vi "Excel Inert Image.vi"(4 "Cell/表格位置2":string, 6 "Cell/表格位置1":string, 8 "错误输入":errorcluster, 9 "图片路径":path, 11 "Excel._Worksheet in":refnum<k7>) -> (0 "错误输出":errorcluster, 2 "AddPicture":refnum<k7>, 3 "Excel._Worksheet out":refnum<k7>)   [LabVIEW 2011]
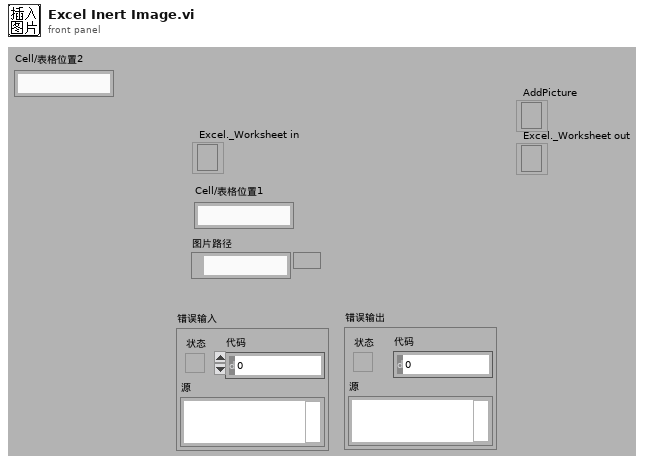
[diagram p1: front panel]
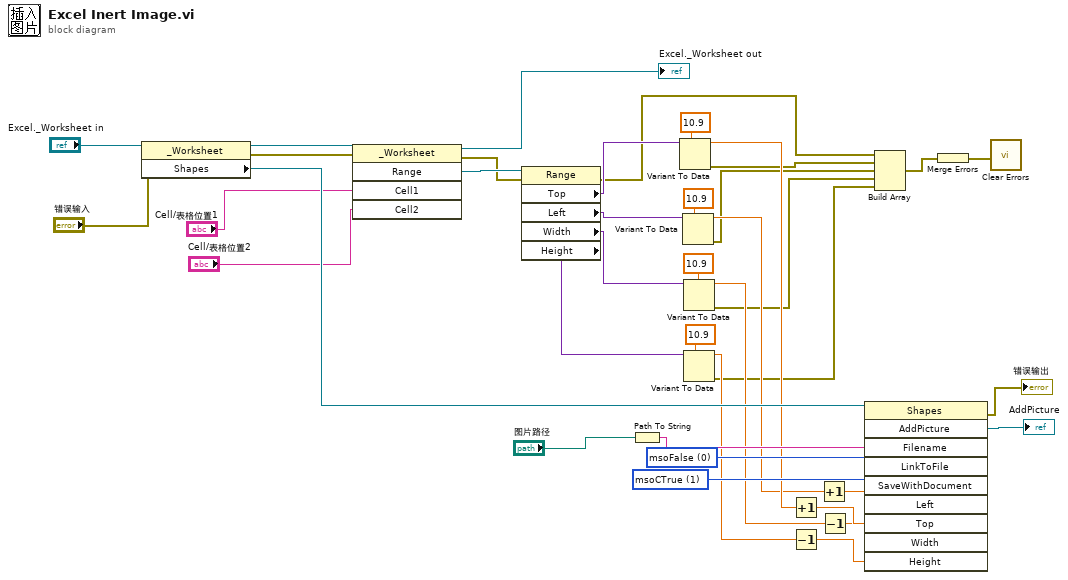
[diagram p0: block diagram]
diagram:
  w33 = 1 items=["msoTrue"=-1, "msoFalse"=0, "msoCTrue"=1, "msoTriStateToggle"=-3, "msoTriStateMixed"=-2] ("SaveWithDocument")
  w34 = 0 items=["msoTrue"=-1, "msoFalse"=0, "msoCTrue"=1, "msoTriStateToggle"=-3, "msoTriStateMixed"=-2] ("LinkToFile")
  n1 = property class="_Worksheet"(reference="Excel._Worksheet in", error in="错误输入") -> (reference out=w39:refnum<k7>, error out=w37:errorcluster, "Shapes"=w38:refnum<k7>)
  n2 = invoke class="_Worksheet" method="Range"(reference=w39, error in=w37, "Cell1"="Cell/表格位置1", "Cell2"="Cell/表格位置2") -> (reference out=→"Excel._Worksheet out":refnum<k7>, error out=w12:errorcluster, "Range"=w26:refnum<k7>)  [unwired: 1 in, 2 out]
  n3 = property class="Range"(reference=w26, error in=w12) -> (error out=w7:errorcluster, "Top"=w25:variant, "Left"=w21:variant, "Width"=w17:variant, "Height"=w15:variant)  [unwired: 1 out]
  n4 = Path To String(path="图片路径") -> (string=w35:string)
  n5 = Variant To Data(type=10.9, Variant=w25) -> (data=w23:dbl, error out=w11:errorcluster)  [unwired: 1 in]
  n6 = Variant To Data(type=10.9, Variant=w21) -> (data=w20:dbl, error out=w10:errorcluster)  [unwired: 1 in]
  n7 = Variant To Data(type=10.9, Variant=w17) -> (data=w16:dbl, error out=w9:errorcluster)  [unwired: 1 in]
  n8 = Variant To Data(type=10.9, Variant=w15) -> (data=w14:dbl, error out=w8:errorcluster)  [unwired: 1 in]
  n9 = Increment(x=w23) -> (x+1=w4:dbl)
  n10 = Decrement(x=w14) -> (x-1=w3:dbl)
  n11 = Increment(x=w20) -> (x+1=w2:dbl)
  n12 = Decrement(x=w16) -> (x-1=w1:dbl)
  n13 = invoke class="Shapes" method="AddPicture"(reference=w38, "Filename"=w35, "LinkToFile"=w34, "SaveWithDocument"=w33, "Left"=w2, "Top"=w4, "Width"=w1, "Height"=w3) -> (error out=→"错误输出":errorcluster, "AddPicture"=→"AddPicture":refnum<k7>)  [unwired: 2 in, 8 out]
  n14 = Build Array(w7, w11, w10, w9, w8) -> (w6:errorcluster[])
  n15 = Merge Errors(w6) -> (w5:errorcluster)
  n16 = call <vilib>:"Clear Errors.vi"("error in (no error)"=w5) -> ()  [unwired: 7 out]
